vi "AWG Write Multiple PreciseRamps.vi"(8 "error in (no error)":errorcluster, 9 "AmpGain":i32=1, 10 "Channel Configurations":T4(array[cluster])=[{"PinNames"=["UP"], "Waveforms Array"=[]}, {"PinNames"=["DOWN"], "Waveforms Array"=[]}] {"Waveforms Array"."Waveform"."Start" min=0.0 max=1.0 format="%.2f"; "Waveforms Array"."Waveform"."End" min=0.0 max=1.0 format="%.2f"}, 11 "Semiconductor Module Context":T1) -> (0 "error out":errorcluster)   [LabVIEW 2013]
uses:
  Utility/PreciseRampWaveformWithName.ctl
  Utility/PreciseRampWaveform.ctl
  <vilib>/NI_TestStand_SemiconductorModule/NI_TestStand_Semiconductor_Module.lvlibp/PinMap/General/SemiconductorModuleContext.ctl
  <instrlib>/niFgen/niFgen.llb/niFgen Write Named Waveform (I16).vi
  <vilib>/NI_TestStand_SemiconductorModule/NI_TestStand_Semiconductor_Module.lvlibp
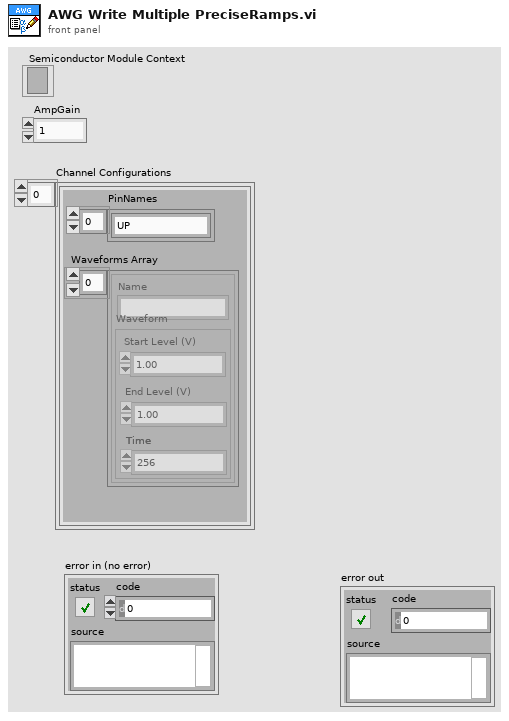
[diagram p1: front panel]
types:
  T1 = typedef "NI_TestStand_Semiconductor_Module.lvlibp/SemiconductorModuleContext.ctl" = refnum<k7>
  T2 = typedef "PreciseRampWaveformWithName.ctl" = cluster{"Name":string, "Waveform":T3}
  T3 = typedef "PreciseRampWaveform.ctl" = cluster{"Start":dbl, "End":dbl, "Time":dbl}
  T4 = cluster{"PinNames":string[], "Waveforms Array":T2[]}[]
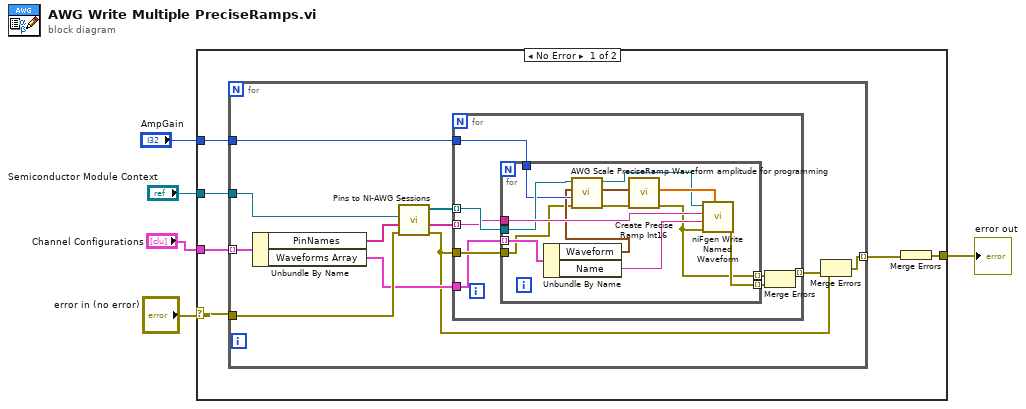
[diagram p0: block diagram]
diagram:
  n1 = case shown="No Error" "error in (no error)" {
    selector: "error in (no error)" -> [w7 w44]
    tunnel: "Channel Configurations" -> [w11 _]
    tunnel: "Semiconductor Module Context" -> [w10 _]
    tunnel: [w8 w44] -> w3
    tunnel: "AmpGain" -> [w6 _]
    frame No Error {
      n2 = for {
        tunnel: [w17] -> w9 mode=indexing
        tunnel: w11 -> [w20] mode=indexing
        tunnel: w7 -> [w19]
        tunnel: w10 -> [w18]
        tunnel: w6 -> [w13]
        n3 = Unbundle By Name(w20) -> ("PinNames"=w15:string[], "Waveforms Array"=w16:T2[])
        n4 = call "Pins to NI-AWG Sessions.vi"("error in (no error)"=w19, "Pins"=w15, "Semiconductor Module Context"=w18) -> ("error out"=w14:errorcluster, "Channel Lists"=w21:string[], "Instrument Sessions"=w22:refnum<k15>[])  [unwired: 5 in, 1 out]
        n5 = for {
          tunnel: w14 -> [w30]
          tunnel: w16 -> [w29]
          tunnel: w22 -> [w26] mode=indexing
          tunnel: w21 -> [w25] mode=indexing
          tunnel: w13 -> [w28]
          tunnel: [w27] -> w12 mode=indexing
          n6 = for {
            tunnel: w30 -> [w35]
            tunnel: w29 -> [w40] mode=indexing
            tunnel: w28 -> [w37]
            tunnel: w26 -> [w38]
            tunnel: w25 -> [w42]
            tunnel: [w41] -> w24 mode=indexing
            tunnel: [w31] -> w23 mode=indexing
            n7 = Unbundle By Name(w40) -> ("Waveform"=w36:T3, "Name"=w33:string)
            n8 = call "AWG Scale PreciseRamp Waveform amplitude for programming.vi"("error in (no error)"=w35, "AmpGain"=w37, "Waveform In"=w36, "Instrument Handle In"=w38) -> ("error out"=w32:errorcluster, "Waveform Out"=w39:T3, "Instrument Handle Out"=w34:refnum<k15>)  [unwired: 5 in]
            n9 = call "Create Precise Ramp Int16.vi"("error in (no error)"=w32, "Waveform"=w39) -> ("error out"=w31:errorcluster, "Waveform Data"=w43:dbl[])  [unwired: 8 in]
            n10 = call-poly <instrlib>:"niFgen Write Named Waveform.vi"("Waveform Data"=w43, "error in (no error)"=w31, "Waveform Name"=w33, "Channel Name"=w42, "Instrument Handle"=w34) -> ("error out"=w41:errorcluster)  [unwired: 4 in, 2 out]
          }
          n11 = Merge Errors(w23, w24) -> (w27:errorcluster)
        }
        n12 = Merge Errors(w14, w12) -> (w17:errorcluster)
      }
      n13 = Merge Errors(w9) -> (w8:errorcluster)
    }
    frame Error {
    }
  }
  "error out" <- w3
